vi "eric's program.vi"   [LabVIEW 2012, in "robot project.lvrbt"]
uses:
  robot project.lvrbt
  <vilib>/FTC/FTC Read Button States.vi
  <vilib>/FTC/FTC Read Controller Packet.vi
  <vilib>/NXT/LegoClasses/BrickReference/BrickReference.lvclass
  <vilib>/NXT/Subs/LVHSConnector.ctl
  <vilib>/NXT/NXTIO Xnodes/NXTIOXNode/NXTIO.xnode
  <vilib>/NXT/Hardware/Plugins/Open Port/OpenPortAddress.ctl
  <vilib>/NXT/NXTIO Xnodes/AddressXNode/NXTIOAddress.xnode
panel:
  # "This VI was generated based on your configuration in the Remote Control Editor. You may modify the code as needed for your robot. To test this program for an FTC match, return to the Remote Control Editor, select the \"Run Program\" tab, and choose \"FTC Game\"."
types:
  T1 = typedef "LVHSConnector.ctl" = refnum<class "BrickReference.lvclass">
  T2 = typedef "FTC ControllerState.ctl" = cluster{"Left X":i8, "Left Y":i8, "Right X":i8, "Right Y":i8, "Button Encoding 9-12":u8, "Button Encoding 1-8":u8, "POV":T3}
  T3 = typedef "FTC POVState.ctl" = i8
  T4 = typedef "FTC ButtonEventType.ctl" = enum16{"Pressed", "Released"}
  T5 = cluster{"Button ID":enum16{"None", "Button 1", "Button 2", "Button 3", "Button 4", "Button 5", "Button 6", "Button 7", "Button 8", "Button 9", "Button 10", "Button 11", "Button 12", "POV Up", "POV Up Right", "POV Right", "POV Down Right", "POV Down", "POV Down Left", "POV Left", "POV Up Left"}, "Event Type":T4}[]
  T6 = enum16{"None", "Button 1", "Button 2", "Button 3", "Button 4", "Button 5", "Button 6", "Button 7", "Button 8", "Button 9", "Button 10", "Button 11", "Button 12", "POV Up", "POV Up Right", "POV Right", "POV Down Right", "POV Down", "POV Down Left", "POV Left", "POV Up Left"}
  T7 = typedef "OpenPortAddress.ctl" = i32
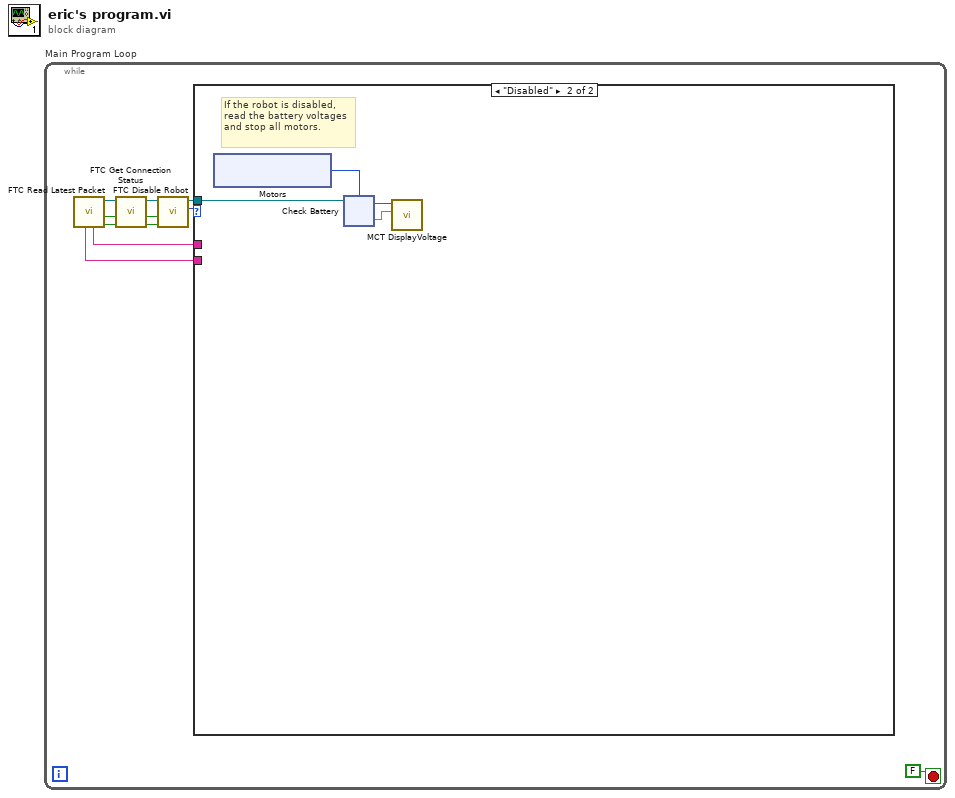
[diagram p0: block diagram]
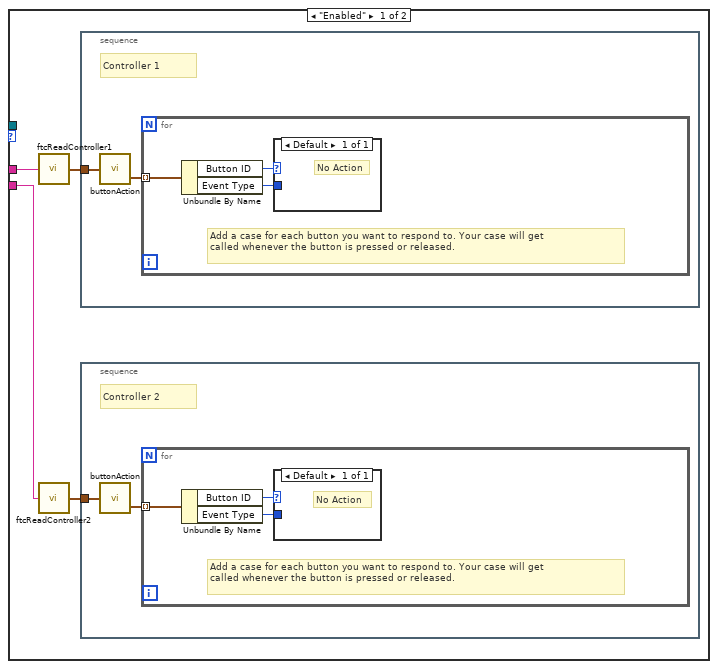
[diagram p2: hidden frame]
diagram:
  n1 = while "Main Program Loop" {
    stop <- FALSE stop-if-true
    n2 = call <vilib>:"FTC Read Latest Packet.vi"() -> ("Packet Received?"=w8:bool, "Stopped?"=w5:bool, "NXT"=w7:T1, "Controller 1"=w10:string, "Controller 2"=w9:string)  [unwired: 6 in, 1 out]
    n3 = call <vilib>:"FTC Get Connection Status.vi"("Packet Received?"=w8, "Stopped?"=w5, "NXT"=w7) -> ("Online?"=w2:bool, "Stopped?"=w3:bool, "NXT"=w4:T1)  [unwired: 5 in]
    n4 = call <vilib>:"FTC Disable Robot.vi"("Online?"=w2, "Stopped?"=w3, "NXT"=w4) -> ("Enabled?"=w6:enum16{"Disabled", "Enabled"}, "NXT"=w1:T1)  [unwired: 3 in]
    n5 = case "disableCase" shown="\"Disabled\"" w6 {
      tunnel: w10 -> [w15 _]
      tunnel: w9 -> [w14 _]
      tunnel: w1 -> [_ w29]
      frame "Enabled" {
        n6 = call "ftcReadController1"("Packet"=w15) -> ("Controller State"=w13:T2)  [unwired: 4 in]
        n7 = call "ftcReadController2"("Packet"=w14) -> ("Controller State"=w12:T2)  [unwired: 4 in]
        n8 = stacked-sequence "controller1Actions" {
          tunnel: w13 -> [w21]
          frame #0 {
            # "Controller 1"
            n9 = call "buttonAction"("Controller State"=w21) -> ("Button Events"=w22:T5)  [unwired: 2 in, 1 out]
            n10 = for "buttonAction" {
              tunnel: w22 -> [w23] mode=indexing
              # "Add a case for each button you want to respond to. Your case will get \ncalled whenever the button is pressed or released."
              n11 = Unbundle By Name(w23) -> ("Button ID"=w25:T6, "Event Type"=w24:T4)
              n12 = case "EventCase1" shown="Default" w25 {
                tunnel: w24 -> [_]
                frame Default {
                  # "No Action"
                }
              }
            }
          }
        }
        n13 = stacked-sequence "controller2Actions" {
          tunnel: w12 -> [w16]
          frame #0 {
            # "Controller 2"
            n14 = call "buttonAction"("Controller State"=w16) -> ("Button Events"=w17:T5)  [unwired: 2 in, 1 out]
            n15 = for "buttonAction" {
              tunnel: w17 -> [w18] mode=indexing
              # "Add a case for each button you want to respond to. Your case will get \ncalled whenever the button is pressed or released."
              n16 = Unbundle By Name(w18) -> ("Button ID"=w20:T6, "Event Type"=w19:T4)
              n17 = case "EventCase2" shown="Default" w20 {
                tunnel: w19 -> [_]
                frame Default {
                  # "No Action"
                }
              }
            }
          }
        }
      }
      frame "Disabled" {
        # "If the robot is disabled, read the battery voltages and stop all motors."
        n18 = xnode ("Motors")() -> ("Motor"=w28:T7)
        n19 = xnode "Check Battery"("Motors"=w28, "NXT"=w29) -> ("Voltage 1"=w27:sgl, "NXT"=w26:T1)
        n20 = call <vilib>:"MCT DisplayVoltage.vi"("Motor Voltage"=w27, "NXT"=w26) -> ()  [unwired: 9 in, 1 out]
      }
    }
  }
